vi "Boiler.vi"() -> ()   [LabVIEW 2020]
uses:
  Controls/Boiler Controls.ctl
  Controls/Boiler Simulation Controls.ctl
  Controls/Boiler Status Indicators.ctl
  Typedefs/ConsumerStates.ctl
  SubVIs/BoilerTimerStates.ctl
panel:
  out "Numeric":i32
  in  "stop":bool
  out "Boiler Status Indicators":T1 {"Time Count" format="%.2g"}
  in  "Boiler Simulation Controls":T2 {"Flame Sensor Value (%)" min=0.0 max=100.0 scale=0.0..100.0}
  in  "Boiler Controls":T3 {"Fuel Valve Position" min=0.0 max=100.0 scale=0.0..100.0 scale format="%.2f"}
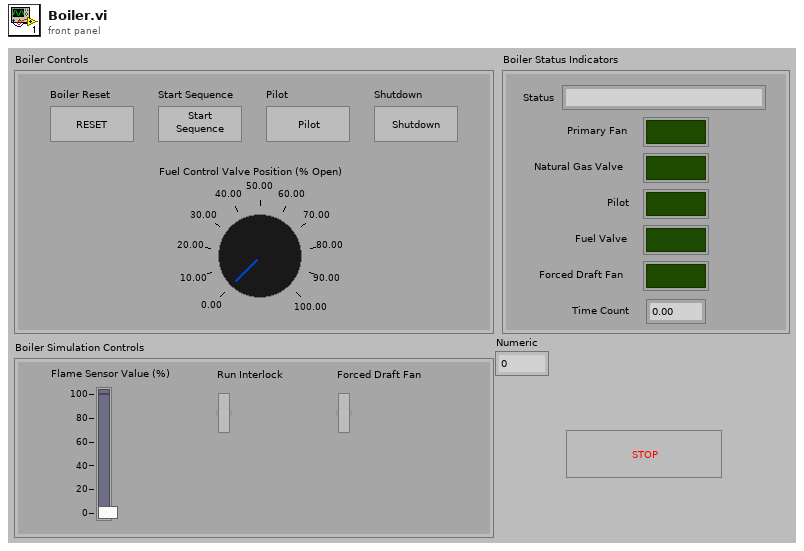
[diagram p1: front panel]
types:
  T1 = typedef "Boiler Status Indicators.ctl" = cluster{"Status":string, "Primary Fan":bool, "Natural Gas Valve":bool, "Pilot":bool, "Fuel Valve":bool, "Forced Draft Fan":bool, "Time Count":dbl}
  T2 = typedef "Boiler Simulation Controls.ctl" = cluster{"Flame Sensor Value (%)":dbl, "Run Interlock":bool, "Forced Draft Fan":bool}
  T3 = typedef "Boiler Controls.ctl" = cluster{"Boiler Reset":bool, "Start Sequence":bool, "Pilot":bool, "Shutdown":bool, "Fuel Valve Position":dbl}
  T4 = typedef "ConsumerStates.ctl" = cluster{"State":enum16{"Idle", "Init", "Reset Lockout", "Start Sequence", "Pilot", "Prove Pilot", "Forced Draft Fan", "Fuel Control Valve", "Boiler Running", "Shutdown", "Error", "Quit"}, "Payload":variant}
  T5 = typedef "BoilerTimerStates.ctl" = enum16{"Start Timer", "Check Timer"}
  T6 = enum16{"Idle", "Init", "Reset Lockout", "Start Sequence", "Pilot", "Prove Pilot", "Forced Draft Fan", "Fuel Control Valve", "Boiler Running", "Shutdown", "Error", "Quit"}
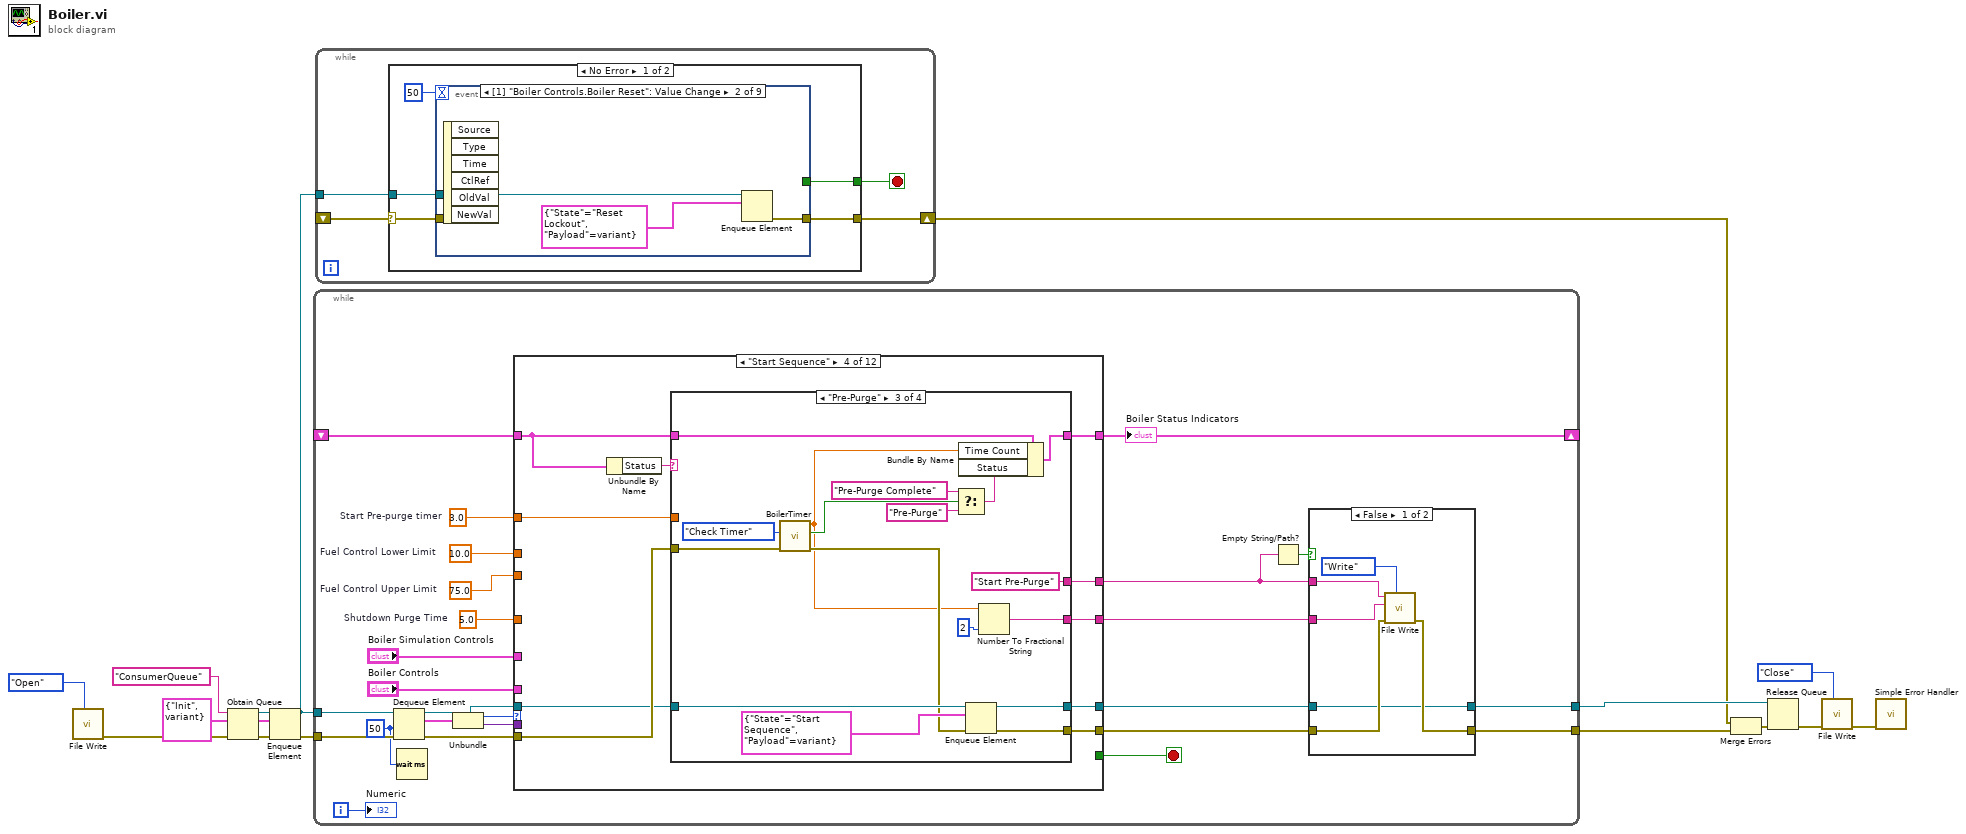
[diagram p0: block diagram]
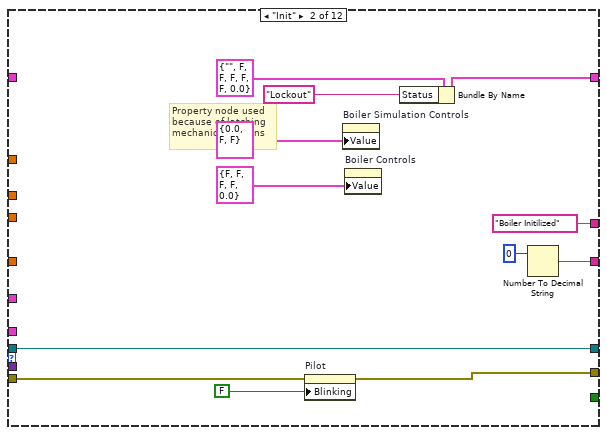
[diagram p4: hidden frame]
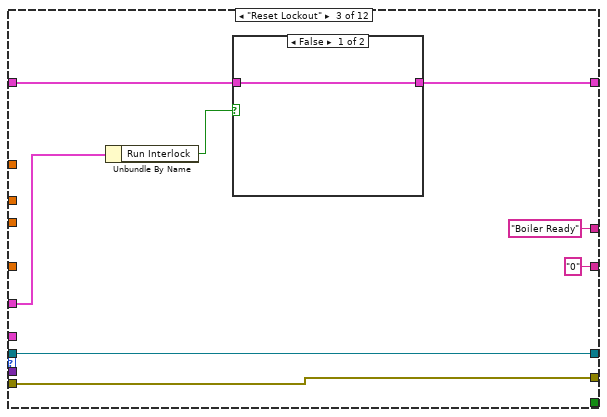
[diagram p5: hidden frame]
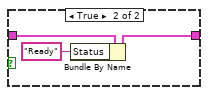
[diagram p6: hidden frame]
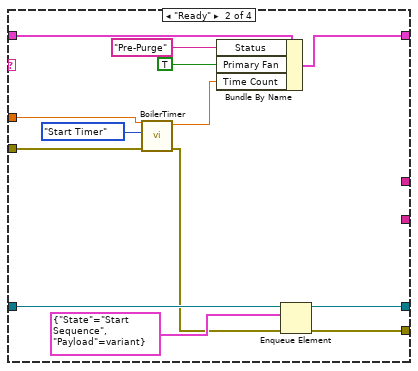
[diagram p8: hidden frame]
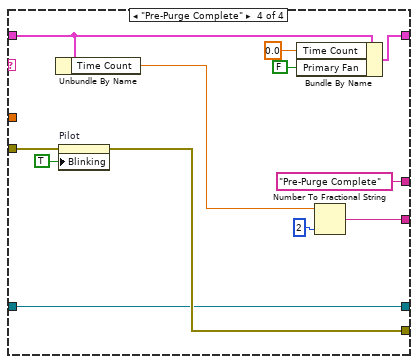
[diagram p9: hidden frame]
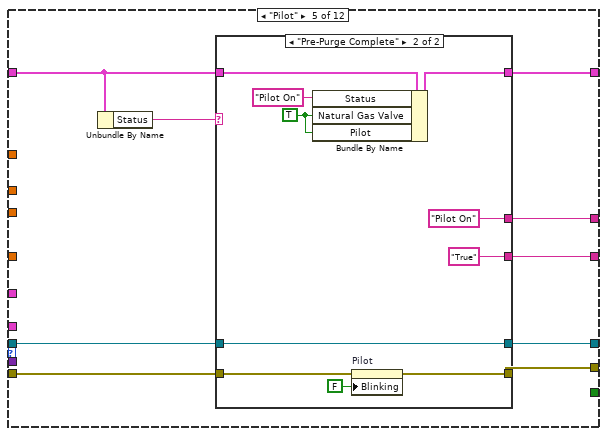
[diagram p10: hidden frame]
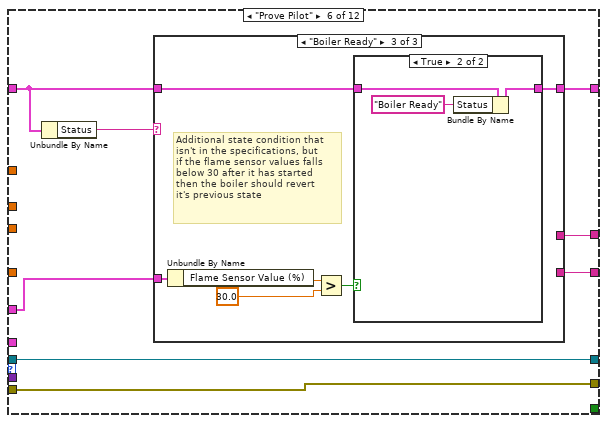
[diagram p12: hidden frame]
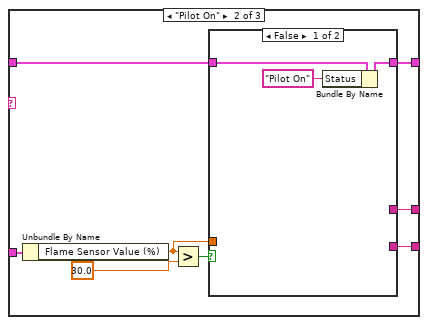
[diagram p14: hidden frame]
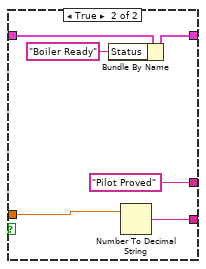
[diagram p15: hidden frame]
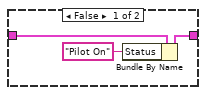
[diagram p16: hidden frame]
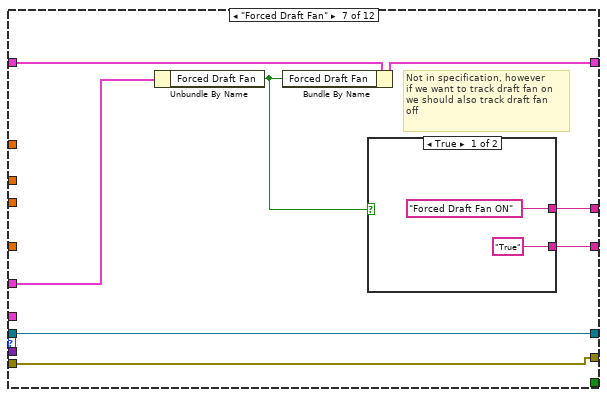
[diagram p17: hidden frame]
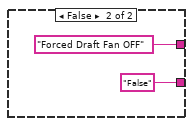
[diagram p18: hidden frame]
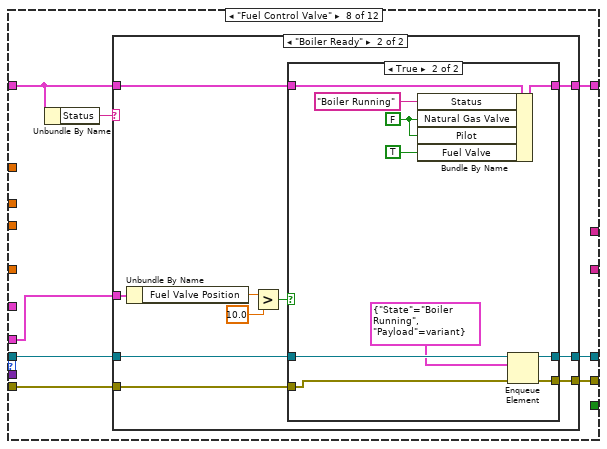
[diagram p19: hidden frame]
diagram:
  w6 = T4 {"State"=enum."Init", "Payload"=variant}
  n1 = call "File Write.vi"("State Control"=enum16{"Open", "Write", "Close"}."Open") -> ("error out"=w3:errorcluster)  [unwired: 10 in]
  n2 = Obtain Queue(name (unnamed)="ConsumerQueue", element data type=w6, error in (no error)=w3) -> (queue out=w11:refnum<queue>, error out=w8:errorcluster)  [unwired: 2 in, 1 out]
  n3 = Enqueue Element(queue=w11, element=w6, error in (no error)=w8) -> (queue out=w9:refnum<queue>, error out=w7:errorcluster)  [unwired: 1 in, 1 out]
  n4 = while {
    tunnel: w7 -> [w39]
    tunnel: w9 -> [w40]
    tunnel: [w18] -> w14
    tunnel: [w21] -> w13
    shift-right: [w33] -> _
    shift-left: _ -> [w32]
    i -> [w27]
    stop <- w35 stop-if-true
    w23 = 3.0  # Start Pre-purge timer
    w24 = 50 ("timeout in ms (-1)")
    w25 = 5.0  # Shutdown Purge Time
    w29 = 75.0  # Fuel Control Upper Limit
    w28 = 10.0  # Fuel Control Lower Limit
    n5 = Dequeue Element(queue=w40, timeout in ms (-1)=w24, error in (no error)=w39) -> (queue out=w26:refnum<queue>, element=w37:T4, error out=w38:errorcluster)  [unwired: 1 out]
    n6 = Wait (ms)(milliseconds to wait=w24) -> ()  [unwired: 1 out]
    n7 = Unbundle(w37) -> ("State"=w36:T6, "Payload"=w34:variant)
    n8 = case shown="\"Start Sequence\"" w36 {
      selector: w36 -> [_ _ _ _ _ _ _ _ _ _ w328 _]
      tunnel: w38 -> [w50 w59 w67 w82 w139 w157 w194 w204 w241 w274 w326 w333]
      tunnel: [_ _ _ _ _ _ _ _ _ _ _ TRUE] -> w35
      tunnel: w34 -> [_ _ _ _ _ _ _ _ _ _ _ _]
      tunnel: [w51 w62 w70 w84 w138 w159 w197 w209 w246 w277 w332 w335] -> w33
      tunnel: "Boiler Simulation Controls" -> [_ _ w69 _ _ w160 w196 _ w252 _ _ _]
      tunnel: "Boiler Controls" -> [_ _ _ _ _ _ _ w210 w253 _ _ _]
      tunnel: w32 -> [w51 _ w71 w85 w137 w156 w198 w208 w246 w276 w332 w335]
      tunnel: w29 -> [_ _ _ _ _ _ _ _ w245 _ _ _]
      tunnel: w28 -> [_ _ _ _ _ _ _ _ w244 _ _ _]
      tunnel: [w49 w55 w66 w79 w134 w158 w195 w205 w242 w272 w325 w334] -> w19
      tunnel: [w50 w56 w67 w81 w133 w157 w194 w203 w240 w270 w326 w333] -> w22
      tunnel: w26 -> [w49 w55 w66 w80 w135 w158 w195 w206 w243 w273 w327 w334]
      tunnel: w25 -> [_ _ _ _ _ _ _ _ _ w271 _ _]
      tunnel: w23 -> [_ _ _ w78 _ _ _ _ _ _ _ _]
      tunnel: [_ w53 "0" w76 w132 w153 w191 _ w238 w268 _ _] -> w20
      tunnel: [_ "Boiler Initilized" "Boiler Ready" w77 w131 w154 w192 _ w239 w269 _ _] -> w17
      frame "Idle" {
        # "Idle case. If no active commands this is called"
      }
      frame "Init" {
        # "Property node used\nbecause of latching\nmechanical actions"
        n9 = property on="Pilot" class="Bool (strict)"(error in=w59, "Blinking"=FALSE) -> (error out=w56:errorcluster)  [unwired: 1 in, 1 out]
        n10 = property on="Boiler Simulation Controls" class="Clust (strict)"("Value"=T2 {"Flame Sensor Value (%)"=0.0, "Run Interlock"=FALSE, "Forced Draft Fan"=FALSE} ("Boiler Simulation Controls")) -> ()  [unwired: 2 in, 2 out]
        n11 = property on="Boiler Controls" class="Clust"("Value"=T3 {"Boiler Reset"=FALSE, "Start Sequence"=FALSE, "Pilot"=FALSE, "Shutdown"=FALSE, "Fuel Valve Position"=0.0} ("Boiler Controls")) -> ()  [unwired: 2 in, 2 out]
        n12 = Bundle By Name(cluster=T1 {"Status"="", "Primary Fan"=FALSE, "Natural Gas Valve"=FALSE, "Pilot"=FALSE, "Fuel Valve"=FALSE, "Forced Draft Fan"=FALSE, "Time Count"=0.0} ("Boiler Status Indicators 2"), "Status"="Lockout") -> (w62:T1)
        n13 = Number To Decimal String(number=0) -> (decimal integer string=w53:string)  [unwired: 1 in]
      }
      frame "Reset Lockout" {
        n14 = Unbundle By Name(w69) -> ("Run Interlock"=w68:bool)
        n15 = case shown="False" w68 {
          tunnel: w71 -> [w72 w75]
          tunnel: [w72 w74] -> w70
          frame False {
          }
          frame True {
            n16 = Bundle By Name(cluster=w75, "Status"="Ready") -> (w74:T1)
          }
        }
      }
      frame "Start Sequence" {
        n17 = Unbundle By Name(w85) -> ("Status"=w83:string)
        n18 = case shown="\"Pre-Purge\"" w83 {
          tunnel: w85 -> [w88 w101 w118 w122]
          tunnel: [w88 w98 w117 w130] -> w84
          tunnel: w82 -> [w87 w97 w116 w127]
          tunnel: [w87 w91 w106 w126] -> w81
          tunnel: w80 -> [w86 w94 w110 w124]
          tunnel: [w86 w90 w109 w124] -> w79
          tunnel: w78 -> [_ w89 _ _]
          tunnel: [_ _ "Start Pre-Purge" "Pre-Purge Complete"] -> w77
          tunnel: [_ _ w103 w121] -> w76
          frame "0", Default {
          }
          frame "Ready" {
            n19 = call "BoilerTimer.vi"("error in (no error)"=w97, "Enum"=BoilerTimerStates."Start Timer", "Timer in"=w89) -> ("error out"=w92:errorcluster, "Elapsed Time"=w95:dbl)  [unwired: 6 in, 1 out]
            n20 = Bundle By Name(cluster=w101, "Status"="Pre-Purge", "Primary Fan"=TRUE, "Time Count"=w95) -> (w98:T1)
            n21 = Enqueue Element(queue=w94, element=T4 {"State"=enum."Start Sequence", "Payload"=variant}, error in (no error)=w92) -> (queue out=w90:refnum<queue>, error out=w91:errorcluster)  [unwired: 1 in, 1 out]
          }
          frame "Pre-Purge" {
            n22 = call "BoilerTimer.vi"("error in (no error)"=w116, "Enum"=BoilerTimerStates."Check Timer") -> ("error out"=w107:errorcluster, "Timer Up"=w113:bool, "Elapsed Time"=w104:dbl)  [unwired: 7 in]
            n23 = Select(t="Pre-Purge Complete", s=w113, f="Pre-Purge") -> (s? t:f=w114:string)
            n24 = Bundle By Name(cluster=w118, "Time Count"=w104, "Status"=w114) -> (w117:T1)
            n25 = Enqueue Element(queue=w110, element=T4 {"State"=enum."Start Sequence", "Payload"=variant}, error in (no error)=w107) -> (queue out=w109:refnum<queue>, error out=w106:errorcluster)  [unwired: 1 in, 1 out]
            n26 = Number To Fractional String(number=w104, precision (6)=i16 2 ("width (-)")) -> (F-format string=w103:string)  [unwired: 2 in]
          }
          frame "Pre-Purge Complete" {
            n27 = Unbundle By Name(w122) -> ("Time Count"=w120:dbl)
            n28 = property on="Pilot" class="Bool (strict)"(error in=w127, "Blinking"=TRUE) -> (error out=w126:errorcluster)  [unwired: 1 in, 1 out]
            n29 = Bundle By Name(cluster=w122, "Time Count"=0.0, "Primary Fan"=FALSE) -> (w130:T1)
            n30 = Number To Fractional String(number=w120, precision (6)=i16 2 ("width (-)")) -> (F-format string=w121:string)  [unwired: 2 in]
          }
        }
      }
      frame "Pilot" {
        n31 = Unbundle By Name(w137) -> ("Status"=w136:string)
        n32 = case shown="\"Pre-Purge Complete\"" w136 {
          tunnel: w137 -> [w142 w152]
          tunnel: w139 -> [w141 w151]
          tunnel: [w141 w150] -> w133
          tunnel: [w142 w148] -> w138
          tunnel: w135 -> [w140 w145]
          tunnel: [w140 w145] -> w134
          tunnel: [_ "True"] -> w132
          tunnel: [_ "Pilot On"] -> w131
          frame "False", Default {
          }
          frame "Pre-Purge Complete" {
            w147 = TRUE ("Natural Gas Valve")
            n33 = Bundle By Name(cluster=w152, "Status"="Pilot On", "Natural Gas Valve"=w147, "Pilot"=w147) -> (w148:T1)
            n34 = property on="Pilot" class="Bool (strict)"(error in=w151, "Blinking"=FALSE) -> (error out=w150:errorcluster)  [unwired: 1 in, 1 out]
          }
        }
      }
      frame "Prove Pilot" {
        n35 = Unbundle By Name(w156) -> ("Status"=w155:string)
        n36 = case shown="\"Boiler Ready\"" w155 {
          tunnel: w160 -> [_ w169 w184]
          tunnel: w156 -> [w161 w168 w183]
          tunnel: [w161 w167 w182] -> w159
          tunnel: [_ w164 _] -> w154
          tunnel: [_ w162 _] -> w153
          frame "False", Default {
            # "If status conditions aren't met do nothing"
          }
          frame "Pilot On" {
            n37 = Unbundle By Name(w169) -> ("Flame Sensor Value (%)"=w163:dbl)
            n38 = Greater?(x=w163, y=30.0) -> (0:w166:bool)
            n39 = case shown="False" w166 {
              tunnel: w168 -> [w172 w178]
              tunnel: [w171 w177] -> w167
              tunnel: [_ "Pilot Proved"] -> w164
              tunnel: w163 -> [_ w174]
              tunnel: [_ w173] -> w162
              frame False {
                n40 = Bundle By Name(cluster=w172, "Status"="Pilot On") -> (w171:T1)
              }
              frame True {
                n41 = Bundle By Name(cluster=w178, "Status"="Boiler Ready") -> (w177:T1)
                n42 = Number To Decimal String(number=w174) -> (decimal integer string=w173:string)  [unwired: 1 in]
              }
            }
          }
          frame "Boiler Ready" {
            # "Additional state condition that \nisn't in the specifications, but\nif the flame sensor values falls\nbelow 30 after it has started\nthen the boiler should revert\nit's previous state"
            n43 = Unbundle By Name(w184) -> ("Flame Sensor Value (%)"=w181:dbl)
            n44 = Greater?(x=w181, y=30.0) -> (0:w180:bool)
            n45 = case shown="True" w180 {
              tunnel: w183 -> [w187 w190]
              tunnel: [w186 w189] -> w182
              frame False {
                n46 = Bundle By Name(cluster=w187, "Status"="Pilot On") -> (w186:T1)
              }
              frame True {
                n47 = Bundle By Name(cluster=w190, "Status"="Boiler Ready") -> (w189:T1)
              }
            }
          }
        }
      }
      frame "Forced Draft Fan" {
        # "Not in specification, however\nif we want to track draft fan on\nwe should also track draft fan\noff"
        n48 = Unbundle By Name(w196) -> ("Forced Draft Fan"=w193:bool)
        n49 = Bundle By Name(cluster=w198, "Forced Draft Fan"=w193) -> (w197:T1)
        n50 = case shown="True" w193 {
          tunnel: ["Forced Draft Fan ON" "Forced Draft Fan OFF"] -> w192
          tunnel: ["True" "False"] -> w191
          frame True {
          }
          frame False {
          }
        }
      }
      frame "Fuel Control Valve" {
        n51 = Unbundle By Name(w208) -> ("Status"=w207:string)
        n52 = case shown="\"Boiler Ready\"" w207 {
          tunnel: w210 -> [_ w223]
          tunnel: w208 -> [w213 w219]
          tunnel: [w213 w218] -> w209
          tunnel: w206 -> [w211 w217]
          tunnel: [w211 w216] -> w205
          tunnel: w204 -> [w212 w215]
          tunnel: [w212 w214] -> w203
          frame "False", Default {
          }
          frame "Boiler Ready" {
            n53 = Unbundle By Name(w223) -> ("Fuel Valve Position"=w221:dbl)
            n54 = Greater?(x=w221, y=10.0) -> (0:w222:bool)
            n55 = case shown="True" w222 {
              tunnel: w219 -> [w226 w236]
              tunnel: [w226 w235] -> w218
              tunnel: w217 -> [w225 w231]
              tunnel: [w225 w230] -> w216
              tunnel: w215 -> [w224 w229]
              tunnel: [w224 w228] -> w214
              frame False {
              }
              frame True {
                w233 = FALSE ("Natural Gas Valve")
                n56 = Bundle By Name(cluster=w236, "Status"="Boiler Running", "Natural Gas Valve"=w233, "Pilot"=w233, "Fuel Valve"=TRUE) -> (w235:T1)
                n57 = Enqueue Element(queue=w231, element=T4 {"State"=enum."Boiler Running", "Payload"=variant}, error in (no error)=w229) -> (queue out=w230:refnum<queue>, error out=w228:errorcluster)  [unwired: 1 in, 1 out]
              }
            }
          }
        }
      }
      frame "Boiler Running" {
        n58 = Unbundle By Name(w253) -> ("Fuel Valve Position"=w237:dbl)
        n59 = Unbundle By Name(w252) -> ("Run Interlock"=w248:bool, "Forced Draft Fan"=w247:bool)
        n60 = Greater?(x=w237, y=w244) -> (0:w250:bool)
        n61 = Less?(x=w237, y=w245) -> (x < y?=w249:bool)
        n62 = Compound Arithmetic op=AND(w250, w249, w248, w247) -> (w251:bool)
        n63 = case shown="True" w251 {
          tunnel: w243 -> [w258 w267]
          tunnel: [w257 w266] -> w242
          tunnel: w241 -> [w255 w265]
          tunnel: [w254 w264] -> w240
          tunnel: [_ "Boiler Running"] -> w239
          tunnel: [_ w260] -> w238
          tunnel: w237 -> [_ w259]
          frame False {
            n64 = Enqueue Element(queue=w258, element=T4 {"State"=enum."Shutdown", "Payload"=variant}, error in (no error)=w255) -> (queue out=w257:refnum<queue>, error out=w254:errorcluster)  [unwired: 1 in, 1 out]
          }
          frame True {
            n65 = Number To Fractional String(number=w259, precision (6)=i16 2 ("width (-)")) -> (F-format string=w260:string)  [unwired: 2 in]
            n66 = Enqueue Element(queue=w267, element=T4 {"State"=enum."Boiler Running", "Payload"=variant}, error in (no error)=w265) -> (queue out=w266:refnum<queue>, error out=w264:errorcluster)  [unwired: 1 in, 1 out]
          }
        }
      }
      frame "Shutdown" {
        n67 = Unbundle By Name(w276) -> ("Status"=w275:string)
        n68 = case shown="\"Lockout\"" w275 {
          tunnel: w276 -> [w280 w298 w302 w323]
          tunnel: [w280 w293 w307 w320] -> w277
          tunnel: w274 -> [w279 w295 w308 w321]
          tunnel: [w279 w288 w308 w312] -> w270
          tunnel: w273 -> [w278 w286 w304 w315]
          tunnel: [w278 w287 w304 w314] -> w272
          tunnel: w271 -> [_ _ _ w316]
          tunnel: [_ "Start Shutdown Purge" "Shutdown Purge Complete" "Start Shutdown Purge"] -> w269
          tunnel: [_ w283 w301 "0"] -> w268
          frame "False", Default {
          }
          frame "Purge" {
            w296 = 10.0  # Purge Time
            n69 = call "BoilerTimer.vi"("error in (no error)"=w295, "Enum"=BoilerTimerStates."Check Timer", "Timer in"=w296) -> ("error out"=w294:errorcluster, "Timer Up"=w289:bool, "Elapsed Time"=w282:dbl)  [unwired: 6 in]
            n70 = Select(t="Lockout", s=w289, f="Purge") -> (s? t:f=w292:string)
            n71 = Bundle By Name(cluster=w298, "Time Count"=w282, "Status"=w292) -> (w293:T1)
            n72 = Enqueue Element(queue=w286, element=T4 {"State"=enum."Shutdown", "Payload"=variant}, error in (no error)=w294) -> (queue out=w287:refnum<queue>, error out=w288:errorcluster)  [unwired: 1 in, 1 out]
            n73 = Number To Decimal String(number=w282, width (-)=i16 2) -> (decimal integer string=w283:string)
          }
          frame "Lockout" {
            w306 = FALSE ("Primary Fan")
            n74 = Unbundle By Name(w302) -> ("Time Count"=w300:dbl)
            n75 = Bundle By Name(cluster=w302, "Primary Fan"=w306, "Natural Gas Valve"=w306, "Pilot"=w306, "Fuel Valve"=w306, "Forced Draft Fan"=w306, "Time Count"=0.0) -> (w307:T1)
            n76 = Number To Decimal String(number=w300, width (-)=i16 2) -> (decimal integer string=w301:string)
          }
          frame "Boiler Running" {
            n77 = call "BoilerTimer.vi"("error in (no error)"=w321, "Enum"=BoilerTimerStates."Start Timer", "Timer in"=w316) -> ("error out"=w313:errorcluster)  [unwired: 6 in, 2 out]
            n78 = Bundle By Name(cluster=w323, "Status"="Purge", "Fuel Valve"=FALSE, "Primary Fan"=TRUE) -> (w320:T1)
            n79 = Enqueue Element(queue=w315, element=T4 {"State"=enum."Shutdown", "Payload"=variant}, error in (no error)=w313) -> (queue out=w314:refnum<queue>, error out=w312:errorcluster)  [unwired: 1 in, 1 out]
          }
        }
      }
      frame "Error", Default {
        n80 = Number To Decimal String(number=w328) -> (decimal integer string=w329:string)  [unwired: 1 in]
        n81 = Concatenate Strings("Undefined Consumer State" ("string"), w329) -> (w330:string)
        n82 = Enqueue Element(queue=w327, element=T4 {"State"=enum."Quit", "Payload"=variant}) -> (queue out=w325:refnum<queue>)  [unwired: 2 in, 2 out]
        n83 = One Button Dialog(message=w330) -> ()  [unwired: 1 in, 1 out]
      }
      frame "Quit" {
      }
    }
    "Boiler Status Indicators" <- w33
    n84 = Empty String/Path?(string/path=w17) -> (empty?=w16:bool)
    n85 = case shown="False" w16 {
      tunnel: w22 -> [w46 w47]
      tunnel: [w45 w47] -> w21
      tunnel: w20 -> [w44 _]
      tunnel: w17 -> [w43 _]
      tunnel: w19 -> [w41 w48]
      tunnel: [w41 w48] -> w18
      frame False {
        n86 = call "File Write.vi"("State Control"=enum16{"Open", "Write", "Close"}."Write", "error in (no error)"=w46, "Event Data String"=w44, "Event String"=w43) -> ("error out"=w45:errorcluster)  [unwired: 7 in]
      }
      frame True {
      }
    }
    "Numeric" <- w27
  }
  n87 = while {
    tunnel: w9 -> [w339]
    shift-right: [w338] -> w5
    shift-left: _ -> [w337]
    stop <- w340 stop-if-true
    n88 = case shown="No Error" w337 {
      selector: w337 -> [w341 w377]
      tunnel: [w345 TRUE ("stop")] -> w340
      tunnel: w339 -> [w344 w375]
      tunnel: [w342 w376] -> w338
      frame No Error {
        n89 = event shown="[1] \"Boiler Controls.Boiler Reset\": Value Change" {
          selector: _ -> [_ _ _ _ _ _ _ _ _]
          dyn-events: _ -> [_ _ _ _ _ _ _ _ _]
          timeout: 50 -> [_ _ _ _ _ _ _ _ _]
          tunnel: [_ _ _ _ _ _ _ _ "stop"] -> w345
          tunnel: w344 -> [_ w348 w351 w354 w357 w360 w363 w366 w371]
          tunnel: [w346 w347 w350 w353 w356 w359 w362 w365 w369] -> w342
          tunnel: w341 -> [w346 _ _ _ _ _ _ _ w368]
          event Timeout {
            n90 = event-data() -> ()  [unwired: 1 in, 3 out]
          }
          event Value Change {
            n91 = event-data() -> ()  [unwired: 1 in, 6 out]
            n92 = Enqueue Element(queue=w348, element=T4 {"State"=enum."Reset Lockout", "Payload"=variant}) -> (error out=w347:errorcluster)  [unwired: 2 in, 2 out]
          }
          event Value Change {
            n93 = event-data() -> ()  [unwired: 1 in, 6 out]
            n94 = Enqueue Element(queue=w351, element=T4 {"State"=enum."Shutdown", "Payload"=variant}) -> (error out=w350:errorcluster)  [unwired: 2 in, 2 out]
          }
          event Value Change {
            n95 = event-data() -> ()  [unwired: 1 in, 6 out]
            n96 = Enqueue Element(queue=w354, element=T4 {"State"=enum."Start Sequence", "Payload"=variant}) -> (error out=w353:errorcluster)  [unwired: 2 in, 2 out]
          }
          event Value Change {
            n97 = event-data() -> ()  [unwired: 1 in, 6 out]
            n98 = Enqueue Element(queue=w357, element=T4 {"State"=enum."Pilot", "Payload"=variant}) -> (error out=w356:errorcluster)  [unwired: 2 in, 2 out]
          }
          event Value Change {
            n99 = event-data() -> ()  [unwired: 1 in, 6 out]
            n100 = Enqueue Element(queue=w360, element=T4 {"State"=enum."Prove Pilot", "Payload"=variant}) -> (error out=w359:errorcluster)  [unwired: 2 in, 2 out]
          }
          event Value Change {
            n101 = event-data() -> ()  [unwired: 1 in, 6 out]
            n102 = Enqueue Element(queue=w363, element=T4 {"State"=enum."Forced Draft Fan", "Payload"=variant}) -> (error out=w362:errorcluster)  [unwired: 2 in, 2 out]
          }
          event Value Change {
            n103 = event-data() -> ()  [unwired: 1 in, 6 out]
            n104 = Enqueue Element(queue=w366, element=T4 {"State"=enum."Fuel Control Valve", "Payload"=variant}) -> (error out=w365:errorcluster)  [unwired: 2 in, 2 out]
          }
          event "stop": Value Change {
            n105 = event-data() -> ()  [unwired: 1 in, 6 out]
            n106 = Enqueue Element(queue=w371, element=T4 {"State"=enum."Quit", "Payload"=variant}, error in (no error)=w368) -> (error out=w369:errorcluster)  [unwired: 1 in, 2 out]
          }
        }
      }
      frame Error {
        n107 = Enqueue Element(queue=w375, element=T4 {"State"=enum."Quit", "Payload"=variant}, error in (no error)=w377) -> (error out=w376:errorcluster)  [unwired: 1 in, 2 out]
      }
    }
  }
  n108 = Merge Errors(w5, w13) -> (w10:errorcluster)
  n109 = Release Queue(queue=w14, error in (no error)=w10) -> (error out=w12:errorcluster)  [unwired: 1 in, 2 out]
  n110 = call "File Write.vi"("State Control"=enum16{"Open", "Write", "Close"}."Close", "error in (no error)"=w12) -> ("error out"=w2:errorcluster)  [unwired: 9 in]
  n111 = call <vilib>:"Simple Error Handler.vi"("error in (no error)"=w2) -> ()  [unwired: 4 in, 5 out]
